vi "GetMotorAngles.vi"(10 "error in (no error)":errorcluster) -> (0 "error out":errorcluster, 1 "Joint3":sgl, 2 "Joint2":sgl, 3 "Joint1":sgl)   [LabVIEW 2013]
uses:
  <vilib>/myRIO/Instrument Drivers/Onboard IO/I2C/vis/Smart Open.vi
  <vilib>/myRIO/Instrument Drivers/Onboard IO/I2C/vis/Configure.vi
  <vilib>/myRIO/Instrument Drivers/Onboard IO/I2C/vis/Write Read.vi
  <vilib>/myRIO/Instrument Drivers/Onboard IO/I2C/vis/Open.vi
  <vilib>/myRIO/Common/Instrument Driver Framework/myRIO v1.0/I2C/vis/myRIO v1.1 Open I2C.vi
  <vilib>/myRIO/Common/Instrument Driver Framework/Utilities/vis/Validate Channels.vi
  <vilib>/myRIO/Common/Instrument Driver Framework/myRIO v1.0/I2C/vis/myRIO v1.0 Reserve I2C.vi
  <vilib>/myRIO/Common/Instrument Driver Framework/myRIO v1.0/I2C/vis/myRIO v1.0 Build MUX Configuration I2C.vi
  <vilib>/myRIO/Common/Instrument Driver Framework/myRIO v1.0/Resource Manager/vis/myRIO v1.0 Reserve Channel List.vi
  <vilib>/myRIO/Common/Instrument Driver Framework/myRIO v1.0/Resource Manager/vis/myRIO v1.0 Create Configuration List.vi
  <vilib>/myRIO/Common/Instrument Driver Framework/myRIO v1.0/Resource Manager/vis/myRIO v1.0 Reserve Channel.vi
  <vilib>/myRIO/Common/Instrument Driver Framework/myRIO v1.0/Resource Manager/vis/myRIO v1.0 Unreserve Channel.vi
  <vilib>/myRIO/Common/Instrument Driver Framework/myRIO v1.0/Resource Manager/vis/myRIO v1.0 Build Mutex Name.vi
  <vilib>/myRIO/Common/Instrument Driver Framework/myRIO v1.0/myRIO v1.1 Open.vi
  <vilib>/Utility/VariantDataType/GetNumericInfo.vi
  <vilib>/Utility/error.llb/Error Cluster From Error Code.vi
  <vilib>/myRIO/Common/Instrument Driver Framework/Utilities/vis/IO Manager.vi
  <vilib>/myRIO/Common/Instrument Driver Framework/Utilities/vis/Configuration Manager.vi
  <vilib>/myRIO/Common/Instrument Driver Framework/myRIO v1.0/Resource Manager/vis/myRIO v1.0 Configure IO.vi
  <vilib>/myRIO/Common/Instrument Driver Framework/myRIO v1.0/myRIO v1.0 Close.vi
  <vilib>/myRIO/Common/Instrument Driver Framework/myRIO v1.0/I2C/vis/myRIO v1.0 Configure I2C.vi
  <vilib>/myRIO/Common/Instrument Driver Framework/myRIO v1.0/I2C/vis/myRIO v1.0 Write I2C.vi
  <vilib>/myRIO/Common/Instrument Driver Framework/myRIO v1.0/I2C/vis/myRIO v1.0 Read I2C.vi
panel:
  out "Long 3":u32 format="%x"
  out "Long 2":u32 format="%x"
  out "Long":u32 format="%x"
  # "hello there"
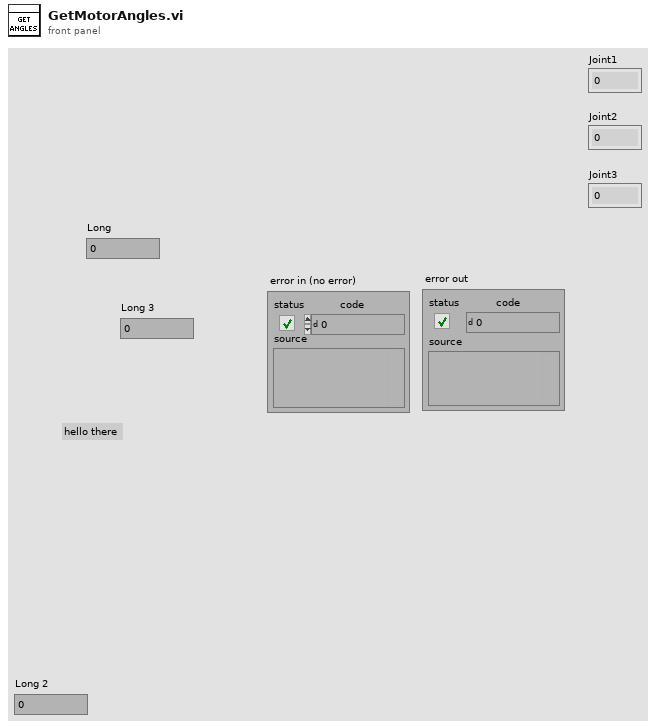
[diagram p1: front panel]
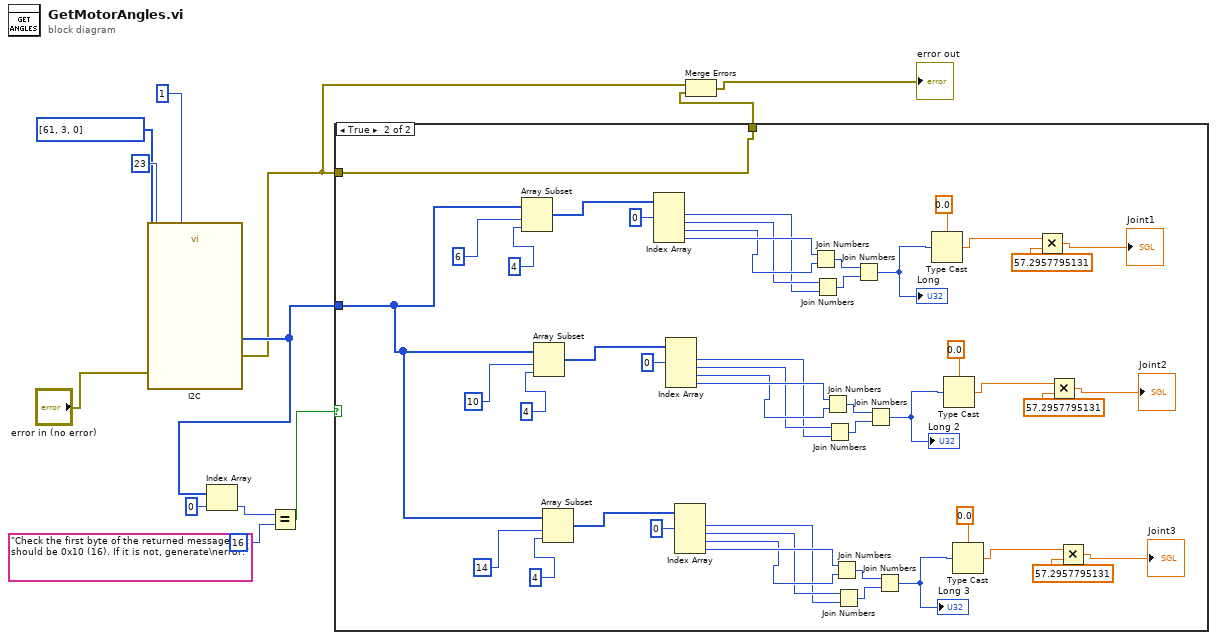
[diagram p0: block diagram]
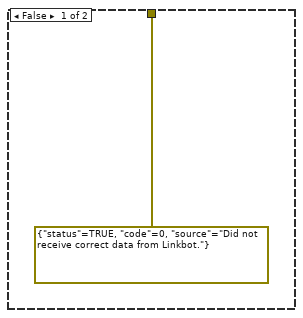
[diagram p2: hidden frame]
diagram:
  (unwired) "Check the first byte of the returned message.\nIt should be 0x10 (16). If it is not, generate\nerror."
  n1 = call "I2C"("Slave Address (7-bit)"=1, "Bytes to Write"=u8[] [61, 3, 0], "Byte Count"=23, "error in (no error)"="error in (no error)") -> ("Bytes Read"=w7:u8[], "error out"=w1:errorcluster)  [unwired: 22 in]
  n2 = Index Array(array=w7, index=0) -> (element=w5:u8)
  n3 = Equal?(x=w5, y=u8 16) -> (x = y?=w3:bool)
  n4 = case shown="True" w3 {
    tunnel: w7 -> [_ w15]
    tunnel: [errorcluster {"status"=TRUE, "code"=0, "source"="Did not receive correct data from Linkbot."} ("error constant") w14] -> w2
    tunnel: w1 -> [_ w14]
    frame False {
    }
    frame True {
      n5 = Array Subset(array=w15, index=6, length=4) -> (w48:u8[])
      n6 = Array Subset(array=w15, index=10, length=4) -> (w33:u8[])
      n7 = Array Subset(array=w15, index=14, length=4) -> (w18:u8[])
      n8 = Index Array(array=w48, index #1=0 ("index")) -> (element #1=w54:u8, element #2=w55:u8, element #3=w56:u8, element #4=w57:u8)  [unwired: 3 in]
      n9 = Index Array(array=w33, index #1=0 ("index")) -> (element #1=w39:u8, element #2=w40:u8, element #3=w41:u8, element #4=w42:u8)  [unwired: 3 in]
      n10 = Index Array(array=w18, index #1=0 ("index")) -> (element #1=w24:u8, element #2=w25:u8, element #3=w26:u8, element #4=w27:u8)  [unwired: 3 in]
      n11 = Join Numbers(hi=w57, lo=w56) -> ((hi.lo)=w51:u16)
      n12 = Join Numbers(hi=w55, lo=w54) -> ((hi.lo)=w52:u16)
      n13 = Join Numbers(hi=w42, lo=w41) -> ((hi.lo)=w36:u16)
      n14 = Join Numbers(hi=w40, lo=w39) -> ((hi.lo)=w37:u16)
      n15 = Join Numbers(hi=w27, lo=w26) -> ((hi.lo)=w21:u16)
      n16 = Join Numbers(hi=w25, lo=w24) -> ((hi.lo)=w22:u16)
      n17 = Join Numbers(hi=w51, lo=w52) -> ((hi.lo)=w50:u32)
      "Long" <- w50
      n18 = Join Numbers(hi=w36, lo=w37) -> ((hi.lo)=w35:u32)
      "Long 2" <- w35
      n19 = Join Numbers(hi=w21, lo=w22) -> ((hi.lo)=w20:u32)
      "Long 3" <- w20
      n20 = Type Cast(type=sgl 0.0, x=w50) -> (*(type *) &x=w58:sgl)
      n21 = Type Cast(type=sgl 0.0, x=w35) -> (*(type *) &x=w43:sgl)
      n22 = Type Cast(type=sgl 0.0, x=w20) -> (*(type *) &x=w28:sgl)
      n23 = Multiply(x=w58, y=57.2957795131) -> (x*y=→"Joint1":dbl)
      n24 = Multiply(x=w43, y=57.2957795131) -> (x*y=→"Joint2":dbl)
      n25 = Multiply(x=w28, y=57.2957795131) -> (x*y=→"Joint3":dbl)
    }
  }
  n26 = Merge Errors(w1, w2) -> (→"error out":errorcluster)
